vi "Get Log Instance.vi"(11 "LoggedActor in":refnum<class "LoggedActor.lvclass">) -> (1 "Log Alias":string, 2 "Log Instance":refnum<class "LoggerReference.lvclass">, 3 "LoggedActor out":refnum<class "LoggedActor.lvclass">)   [LabVIEW 2019, in "LoggedActor.lvclass"]
uses:
  <vilib>/gpm_packages/@cs/Network-interface/Source/Logged Actor/LoggedActor.lvclass
  <vilib>/gpm_packages/@cs/event-logger/Source/Composed Log/LoggerReference/LoggerReference.lvclass
  <vilib>/gpm_packages/@cs/Network-interface/Source/Logged Actor/LoggedActor.lvclass/LoggedActor.ctl
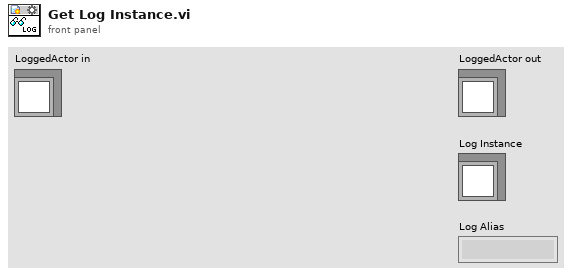
[diagram p1: front panel]
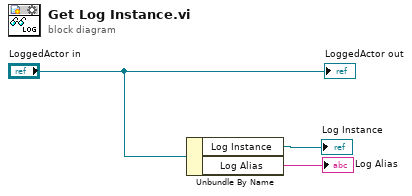
[diagram p0: block diagram]
diagram:
  n1 = Unbundle By Name("LoggedActor in") -> ("Log Instance"=→"Log Instance":refnum<class "LoggerReference.lvclass">, "Log Alias"=→"Log Alias":string)
  "LoggedActor out" <- "LoggedActor in"
